vi "Obtain System Ref.vi"(8 "error in (no error)":errorcluster) -> (0 "error out":errorcluster, 3 "JKI SMO System":refnum<data-value>)   [LabVIEW 2019, in "Registry-SMO.lvclass"]
doc: "JKI State Machine Objects (SMO) 1.3.0.56\nJKI - JKI\nCopyright (c) 2017, JKI"
uses:
  Registry-SMO.lvclass
  SMO_Info--Cluster.ctl
  Registry-SMO.lvclass/Registry-SMO.ctl
  Support/Attribute.Identity/Attribute.Identity.lvclass
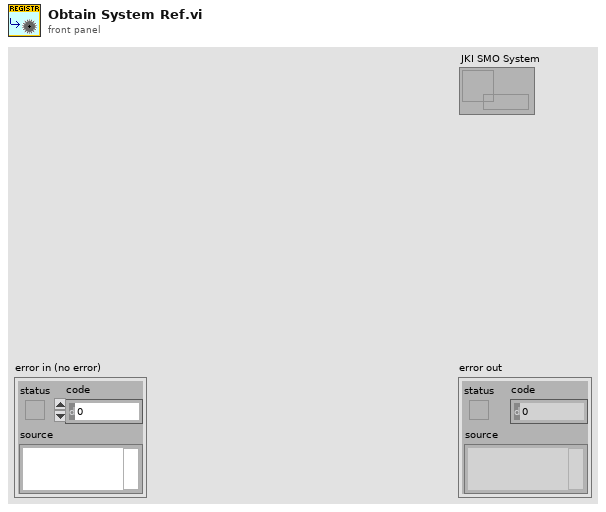
[diagram p1: front panel]
types:
  T1 = typedef "Registry-SMO.lvclass/SMO_Info--Cluster.ctl" = cluster{"Name":string, "Shared Resource":bool}
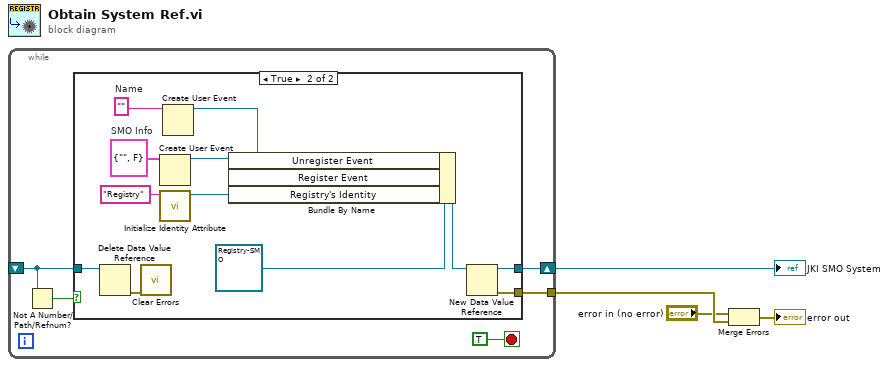
[diagram p0: block diagram]
diagram:
  n1 = while {
    shift-right: [w9] -> w4
    shift-left: _ -> [w6]
    tunnel: [w5] -> w3
    stop <- TRUE stop-if-true
    n2 = Not A Number/Path/Refnum?(number/path/refnum=w6) -> (NaN/Path/Refnum?=w7:bool)
    n3 = case shown="True" w7 {
      tunnel: [w10 w22] -> w9
      tunnel: w6 -> [w10 w12]
      tunnel: [_ w21] -> w5
      frame False {
      }
      frame True {
        w14 = ""  # Name
        w19 = T1 {"Name"="", "Shared Resource"=FALSE}  # SMO Info
        n4 = Delete Data Value Reference(data value reference=w12) -> (error out=w11:errorcluster)  [unwired: 1 in, 1 out]
        n5 = call <vilib>:"Clear Errors.vi"("error in (no error)"=w11) -> ()  [unwired: 5 in, 2 out]
        n6 = Create User Event(user event datatype=w19) -> (user event=w15:refnum<user-event>)  [unwired: 1 in, 1 out]
        n7 = call "Initialize Identity Attribute.vi"("Name"="Registry") -> ("Attribute.Identity"=w18:refnum<class "Attribute.Identity.lvclass">)  [unwired: 10 in]
        n8 = Create User Event(user event datatype=w14) -> (user event=w13:refnum<user-event>)  [unwired: 1 in, 1 out]
        n9 = Bundle By Name(cluster=refnum<class "Registry-SMO.lvclass"> refnum ("JKI SMO System"), "Unregister Event"=w13, "Register Event"=w15, "Registry's Identity"=w18) -> (w16:refnum<class "Registry-SMO.lvclass">)
        n10 = New Data Value Reference(data value=w16) -> (data value reference=w22:refnum<data-value>, error out=w21:errorcluster)  [unwired: 1 in]
      }
    }
  }
  "JKI SMO System" <- w4
  n11 = Merge Errors("error in (no error)", w3) -> (→"error out":errorcluster)
